vi "MCLB StrEdit Resize.vi"(8 "error in (no error)":errorcluster, 11 "View in":refnum<class "MCListbox View.lvclass">) -> (0 "error out":errorcluster, 3 "View out":refnum<class "MCListbox View.lvclass">)   [LabVIEW 2013, in "SET Project Editor.lvlib" / "MCListbox View.lvclass"]
uses:
  MCListbox View.lvclass
  <vilib>/Utility/miscctls.llb/LVBoundsTypeDef.ctl
  MCListbox View.lvclass/MCListbox View.ctl
  Lib/Unicode/SET_Unicode Tools.lvlib
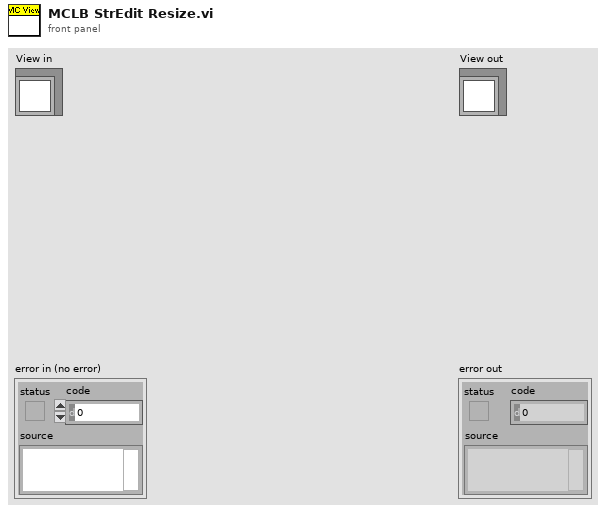
[diagram p1: front panel]
types:
  T1 = typedef "LVBoundsTypeDef.ctl" = cluster{"Width":u32, "Height":u32}
  T2 = typedef "LVRowAndColumnTypeDef.ctl" = cluster{"Row":i32, "Column":i32}
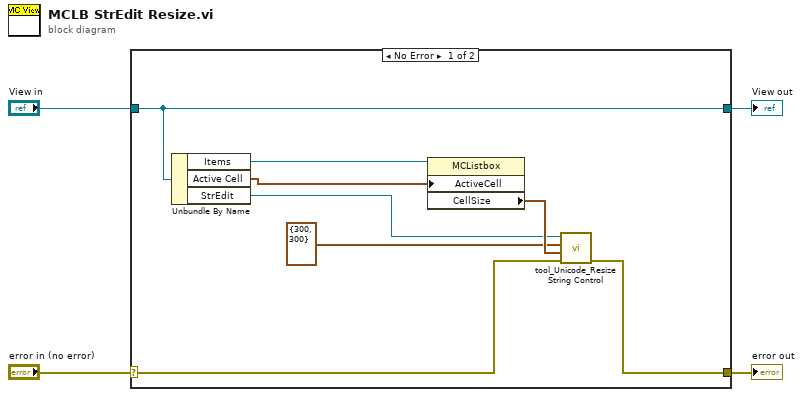
[diagram p0: block diagram]
diagram:
  n1 = case shown="No Error" "error in (no error)" {
    selector: "error in (no error)" -> [w7 w14]
    tunnel: [w6 w14] -> w3
    tunnel: [w5 w13] -> w1
    tunnel: "View in" -> [w5 w13]
    frame No Error {
      n2 = Unbundle By Name(w5) -> ("Items"=w11:refnum<vi>, "Active Cell"=w10:T2, "StrEdit"=w8:refnum<vi>)
      n3 = property class="MCListbox"(reference=w11, "ActiveCell"=w10) -> ("CellSize"=w12:T1)  [unwired: 1 in, 2 out]
      n4 = call "tool_Unicode_Resize String Control.vi"("error in (no error)"=w7, "Min Size (10x10)"=w12, "Max Size (300x300)"=T1 {"Width"=300, "Height"=300}, "*StrControl in"=w8) -> ("error out"=w6:errorcluster)  [unwired: 6 in, 1 out]
    }
    frame Error {
    }
  }
  "error out" <- w3
  "View out" <- w1
